vi "$String to Numeric.vi"(11 "Amount Deposited In":string) -> (2 "Amount":dbl, 3 "Amount Deposited Out":string)   [LabVIEW 2020]
doc: "This VI Reads and increments the \"Amount Deposited\""
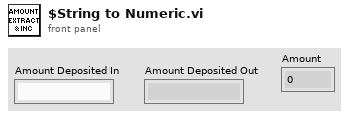
[diagram p1: front panel]
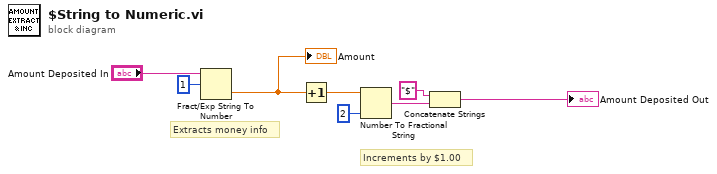
[diagram p0: block diagram]
diagram:
  # "Increments by $1.00"
  # "Extracts money info"
  n1 = Fract/Exp String To Number(string="Amount Deposited In", offset=1) -> (number=w1:dbl)  [unwired: 2 in, 1 out]
  "Amount" <- w1
  n2 = Increment(x=w1) -> (x+1=w2:dbl)
  n3 = Number To Fractional String(number=w2, precision (6)=i16 2) -> (F-format string=w4:string)  [unwired: 2 in]
  n4 = Concatenate Strings("$" ("string"), w4) -> (→"Amount Deposited Out":string)
